vi "Serialization Test.vi"() -> ()   [LabVIEW 2014, in "Modbus Tests.lvlib"]
uses:
  Modbus Tests.lvlib
  module/configuration/Modbus Module configuration.lvclass
panel:
  out "modules equal":bool
  out "channels equal":bool
  out "error in":errorcluster
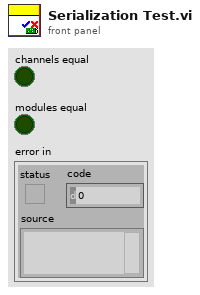
[diagram p1: front panel]
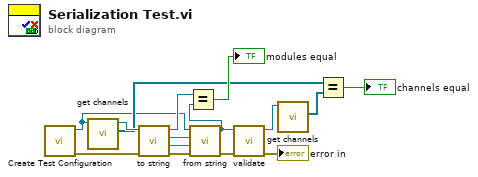
[diagram p0: block diagram]
diagram:
  n1 = call "Create Test Configuration.vi"() -> ("error out"=w2:errorcluster, "Module configuration"=w4:refnum<class "Modbus Module configuration.lvclass">)  [unwired: 9 in, 1 out]
  n2 = call-dynamic "get channels.vi"("Modbus Slave configuration in"=w4) -> ("channels"=w6:refnum<class "TBM channel.lvclass">[], "Modbus Slave configuration out"=w7:refnum<class "Modbus Module configuration.lvclass">)  [unwired: 9 in]
  n3 = call-dynamic "to string.vi"("error in"=w2, "Modbus Slave configuration in"=w7) -> ("error out"=w15:errorcluster, "data"=w14:string, "version"=w13:string, "Modbus Slave configuration out"=w5:refnum<class "Modbus Module configuration.lvclass">)  [unwired: 6 in]
  n4 = call-dynamic "from string.vi"("error in"=w15, "data"=w14, "version"=w13, "Modbus Slave configuration in"=w4) -> ("error out"=w12:errorcluster, "Modbus Slave configuration out"=w1:refnum<class "Modbus Module configuration.lvclass">)  [unwired: 6 in]
  n5 = Equal?(x=w5, y=w1) -> (x = y?=→"modules equal":bool)
  n6 = call-dynamic "validate.vi"("error in"=w12, "Modbus Slave configuration in"=w1) -> ("error out"=→"error in":errorcluster, "Modbus Slave configuration out"=w10:refnum<class "Modbus Module configuration.lvclass">)  [unwired: 8 in]
  n7 = call-dynamic "get channels.vi"("Modbus Slave configuration in"=w10) -> ("channels"=w9:refnum<class "TBM channel.lvclass">[])  [unwired: 9 in, 1 out]
  n8 = Equal?(x=w6, y=w9) -> (x = y?=→"channels equal":bool)
